vi "Main.vi"() -> ()   [LabVIEW 2018]
uses:
  Mul.vi
panel:
  in  "stop":bool
  out "C":dbl
  in  "B":dbl
  in  "A":dbl
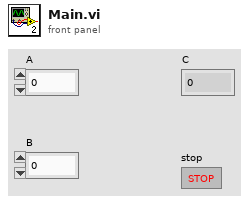
[diagram p1: front panel]
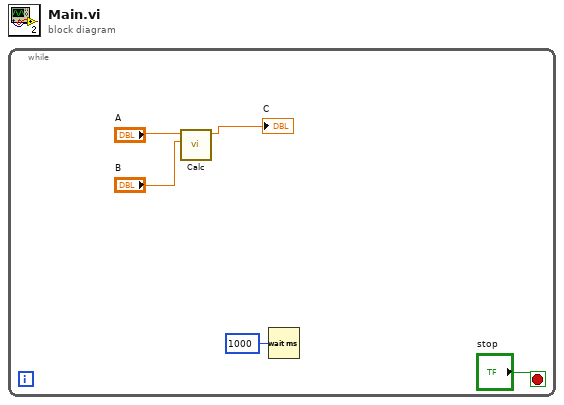
[diagram p0: block diagram]
diagram:
  n1 = while {
    stop <- "stop" stop-if-true
    n2 = call-poly "Calc.vi"("B"="B", "A"="A") -> ("C"=→"C":dbl)  [unwired: 9 in]
    n3 = Wait (ms)(milliseconds to wait=u32 1000) -> ()  [unwired: 1 out]
  }
